vi "JSONRPC-InvokeMethod.vi"(7 "method":T1(ring), 8 "error in (no error)":errorcluster, 11 "params":string[](array[string])) -> (0 "error out":errorcluster, 3 "result":string)   [LabVIEW 2015]
doc: "Invokes the actual implementation of a RIP <b>method</b>."
uses:
  JSONRPC-GetAsString.vi
  JSONRPC-ArrayToString_Cluster.vi
  Configuration/Global_Configurations.vi
  JSONRPC-ArrayToString_String.vi
  JSONRPC-GetAsArray.vi
panel:
  # "InvokeMethod"
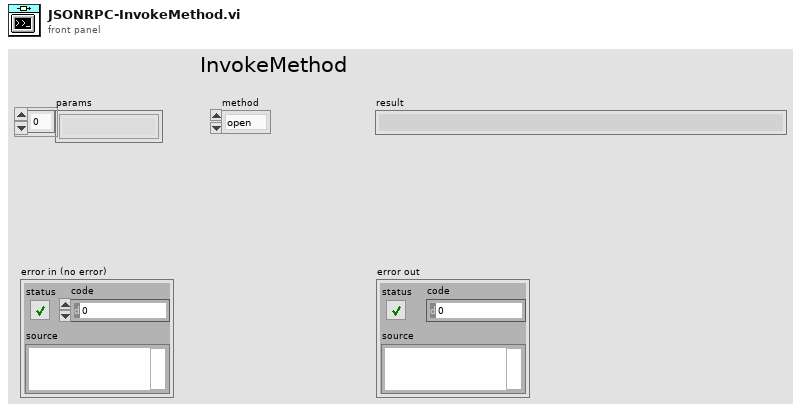
[diagram p1: front panel]
types:
  T1 = enum16{"open", "close", "start", "stop", "get", "set", "info", "UNDEFINED"}
  T2 = enum16{"Parse error", "Invalid request", "Method not found", "Invalid params", "Internal error", "Server error", ""}
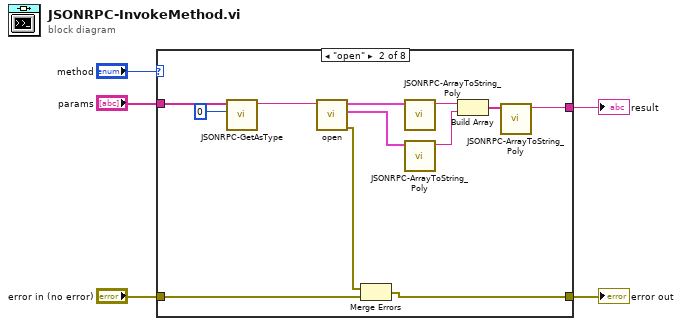
[diagram p0: block diagram]
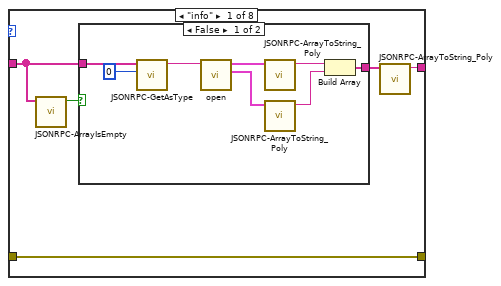
[diagram p2: hidden frame]
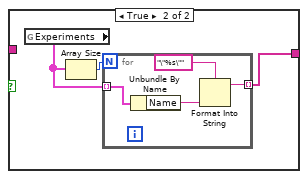
[diagram p3: hidden frame]
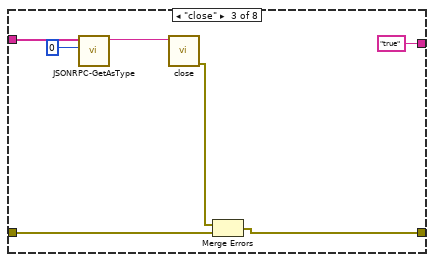
[diagram p4: hidden frame]
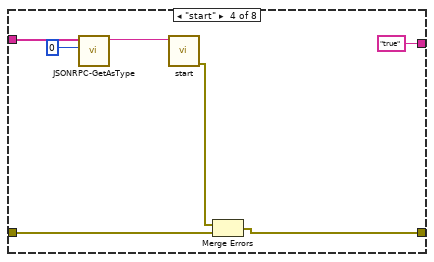
[diagram p5: hidden frame]
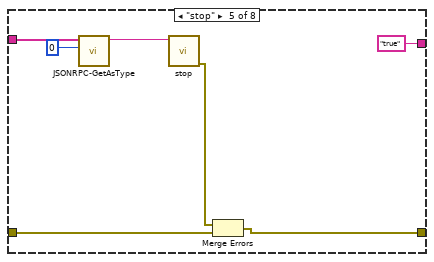
[diagram p6: hidden frame]
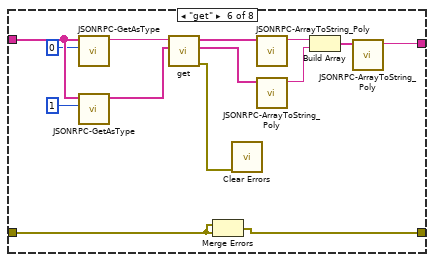
[diagram p7: hidden frame]
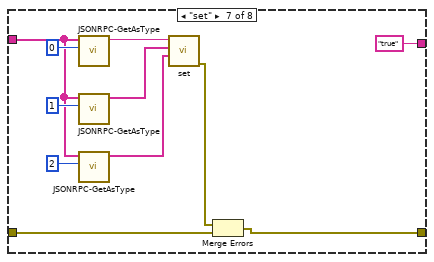
[diagram p8: hidden frame]
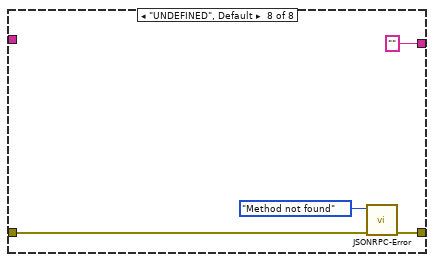
[diagram p9: hidden frame]
diagram:
  n1 = case shown="\"open\"" "method" {
    tunnel: "params" -> [w9 w30 w38 w45 w54 w66 w74 _]
    tunnel: [w7 w28 "true" "true" "true" w61 "true" ""] -> w2
    tunnel: [w10 w36 w41 w48 w55 w72 w80 w86] -> w3
    tunnel: "error in (no error)" -> [w10 w37 w42 w49 w56 w60 w81 w84]
    frame "info" {
      n2 = call "JSONRPC-ArrayIsEmpty.vi"("input array"=w9) -> ("empty?"=w8:bool)  [unwired: 10 in]
      n3 = case shown="False" w8 {
        tunnel: w9 -> [w17 _]
        tunnel: [w11 w19] -> w6
        frame False {
          n4 = call-poly "JSONRPC-GetAsType.vi"("index"=0, "params"=w17) -> ("output"=w16:string)  [unwired: 9 in]
          n5 = call "open.vi"("Experience ID"=w16) -> ("Controls_list"=w12:cluster{"Name":string, "Type":string}[], "Indicators_list"=w13:cluster{"Name":string, "Type":string}[])  [unwired: 8 in, 1 out]
          n6 = call-poly "JSONRPC-ArrayToString_Poly.vi"("Array"=w13) -> ("Output"=w14:string)  [unwired: 10 in]
          n7 = call-poly "JSONRPC-ArrayToString_Poly.vi"("Array"=w12) -> ("Output"=w15:string)  [unwired: 10 in]
          n8 = Build Array(w14, w15) -> (w11:string[])
        }
        frame True {
          n9 = global read "Global_Configurations.vi" "Experiments"() -> (w20:cluster{"Path":path, "Name":string}[])
          n10 = Array Size(array=w20) -> (size(s)=w21:i32)
          n11 = for {
            N: w21 -> [_]
            tunnel: w20 -> [w25] mode=indexing
            tunnel: [w22] -> w19 mode=indexing
            n12 = Unbundle By Name(w25) -> ("Name"=w24:string)
            n13 = Format Into String(format string="\"%s\"", w24) -> (resulting string=w22:string)  [unwired: 2 in, 1 out]
          }
        }
      }
      n14 = call-poly "JSONRPC-ArrayToString_Poly.vi"("Array"=w6) -> ("Output"=w7:string)  [unwired: 10 in]
    }
    frame "open" {
      n15 = call-poly "JSONRPC-GetAsType.vi"("index"=0, "params"=w30) -> ("output"=w31:string)  [unwired: 9 in]
      n16 = call "open.vi"("Experience ID"=w31) -> ("error out"=w35:errorcluster, "Controls_list"=w26:cluster{"Name":string, "Type":string}[], "Indicators_list"=w27:cluster{"Name":string, "Type":string}[])  [unwired: 8 in]
      n17 = Merge Errors(w35, w37) -> (w36:errorcluster)
      n18 = call-poly "JSONRPC-ArrayToString_Poly.vi"("Array"=w27) -> ("Output"=w29:string)  [unwired: 10 in]
      n19 = call-poly "JSONRPC-ArrayToString_Poly.vi"("Array"=w26) -> ("Output"=w34:string)  [unwired: 10 in]
      n20 = Build Array(w29, w34) -> (w33:string[])
      n21 = call-poly "JSONRPC-ArrayToString_Poly.vi"("Array"=w33) -> ("Output"=w28:string)  [unwired: 10 in]
    }
    frame "close" {
      n22 = call-poly "JSONRPC-GetAsType.vi"("index"=0, "params"=w38) -> ("output"=w39:string)  [unwired: 9 in]
      n23 = call "close.vi"("Experience ID"=w39) -> ("error out"=w43:errorcluster)  [unwired: 10 in]
      n24 = Merge Errors(w43, w42) -> (w41:errorcluster)
    }
    frame "start" {
      n25 = call-poly "JSONRPC-GetAsType.vi"("index"=0, "params"=w45) -> ("output"=w46:string)  [unwired: 9 in]
      n26 = call "start.vi"("Experience ID"=w46) -> ("error out"=w50:errorcluster)  [unwired: 10 in]
      n27 = Merge Errors(w50, w49) -> (w48:errorcluster)
    }
    frame "stop" {
      n28 = call-poly "JSONRPC-GetAsType.vi"("index"=0, "params"=w54) -> ("output"=w52:string)  [unwired: 9 in]
      n29 = call "stop.vi"("Experience ID"=w52) -> ("error out"=w57:errorcluster)  [unwired: 10 in]
      n30 = Merge Errors(w57, w56) -> (w55:errorcluster)
    }
    frame "get" {
      n31 = call-poly "JSONRPC-GetAsType.vi"("index"=0, "params"=w66) -> ("output"=w62:string)  [unwired: 9 in]
      n32 = call-poly "JSONRPC-GetAsType.vi"("index"=1, "params"=w66) -> ("output"=w63:string[])  [unwired: 9 in]
      n33 = call "get.vi"("variables"=w63, "Experience ID"=w62) -> ("error out"=w59:errorcluster, "values"=w70:string[], "names"=w68:string[])  [unwired: 7 in]
      n34 = Merge Errors(w60, w60) -> (w72:errorcluster)
      n35 = call <vilib>:"Clear Errors.vi"("error in (no error)"=w59) -> ()  [unwired: 5 in, 2 out]
      n36 = call-poly "JSONRPC-ArrayToString_Poly.vi"("Array"=w68) -> ("Output"=w67:string)  [unwired: 10 in]
      n37 = call-poly "JSONRPC-ArrayToString_Poly.vi"("Array"=w70) -> ("Output"=w71:string)  [unwired: 10 in]
      n38 = Build Array(w67, w71) -> (w69:string[])
      n39 = call-poly "JSONRPC-ArrayToString_Poly.vi"("Array"=w69) -> ("Output"=w61:string)  [unwired: 10 in]
    }
    frame "set" {
      n40 = call-poly "JSONRPC-GetAsType.vi"("index"=0, "params"=w74) -> ("output"=w79:string)  [unwired: 9 in]
      n41 = call-poly "JSONRPC-GetAsType.vi"("index"=1, "params"=w74) -> ("output"=w77:string[])  [unwired: 9 in]
      n42 = call-poly "JSONRPC-GetAsType.vi"("index"=2, "params"=w74) -> ("output"=w73:string[])  [unwired: 9 in]
      n43 = call "set.vi"("values"=w73, "variables"=w77, "Experience ID"=w79) -> ("error out"=w82:errorcluster)  [unwired: 8 in]
      n44 = Merge Errors(w82, w81) -> (w80:errorcluster)
    }
    frame "UNDEFINED", Default {
      n45 = call "JSONRPC-Error.vi"("error in"=w84, "Type"=T2."Method not found") -> ("error out"=w86:errorcluster)  [unwired: 9 in]
    }
  }
  "error out" <- w3
  "result" <- w2
